vi "Configure Additional PUSCH Allocation.vi"(0 "VISA resource name":refnum<visa-resource-name>, 1 "DMRS Length (1)":i32=1, 2 "DMRS Power (0.0)":dbl format="%^.3e", 5 "Instance (1)":T3=1, 7 "Carrier Component (1)":T2=1, 9 "Allocation (1)":T1=1, 11 "error in (no error)":errorcluster, 12 "CDM Groups (1)":i32=1, 13 "Antenna Port (0)":i32) -> (4 "VISA resource name out":refnum<visa-resource-name>, 15 "error out":errorcluster)   [LabVIEW 2015, in "Rohde&Schwarz CMXP NR FR2 Measurement.lvlib"]
doc: "Specifies settings related to the PUSCH allocation, for carrier <no>, allocation <a>.\n\nAttribute:\nRSCMXPNRFR2M_ATTR_ADDITIONAL_PUSCH_ALLOCATION\n\nRemote-control command:\nCONFigure:NRMMw:MEAS<i>[:CC<no>]:ALLocation<a>:PUSCh:ADDitional"
uses:
  <instrlib>/Rohde&Schwarz CMXP NR FR2 Measurement/Rohde&Schwarz CMXP NR FR2 Measurement.lvlib
  <instrlib>/Rohde&Schwarz CMXP NR FR2 Measurement/Private/_Instance.ctl
  <instrlib>/Rohde&Schwarz CMXP NR FR2 Measurement/Private/_Carrier Component.ctl
  <instrlib>/Rohde&Schwarz CMXP NR FR2 Measurement/Private/_Allocation.ctl
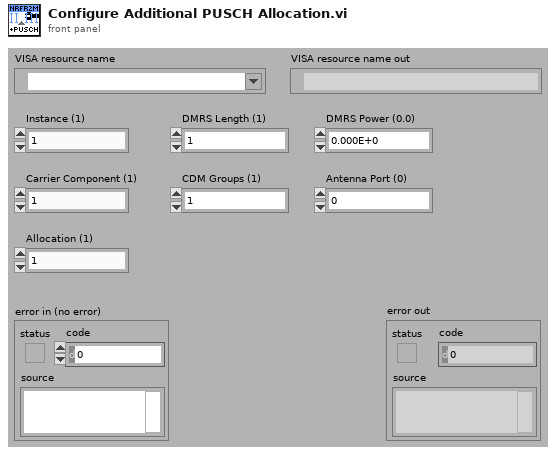
[diagram p1: front panel]
types:
  T1 = typedef "Rohde&Schwarz CMXP NR FR2 Measurement.lvlib/_Allocation.ctl" = i32
  T2 = typedef "Rohde&Schwarz CMXP NR FR2 Measurement.lvlib/_Carrier Component.ctl" = i32
  T3 = typedef "Rohde&Schwarz CMXP NR FR2 Measurement.lvlib/_Instance.ctl" = i32
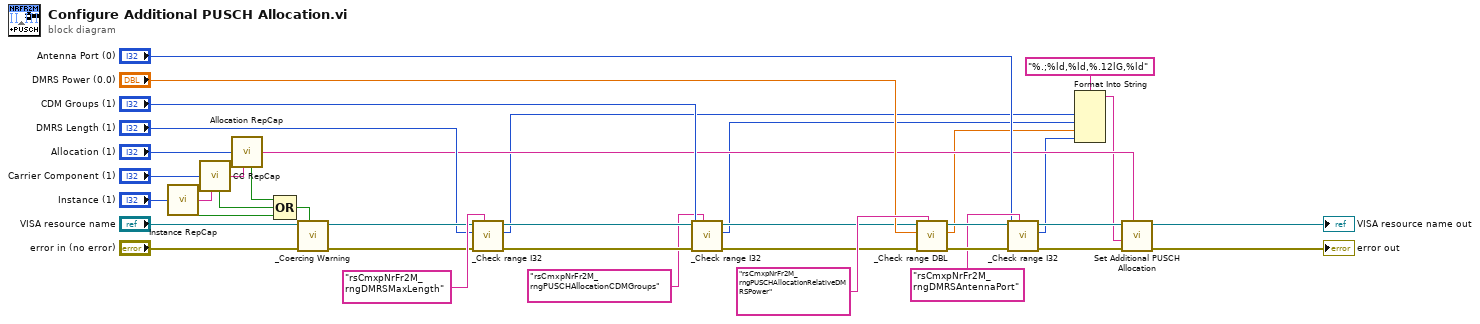
[diagram p0: block diagram]
diagram:
  n1 = call <instrlib>:"Instance RepCap.vi"("Instance In"="Instance (1)") -> ("In Range?"=w34:bool, "RepCap Identifier Out"=w2:string)  [unwired: 1 in]
  n2 = call <instrlib>:"CC RepCap.vi"("CC In"="Carrier Component (1)", "RepCap String In (\"\")"=w2) -> ("In Range?"=w33:bool, "RepCap Identifier Out"=w32:string)
  n3 = call <instrlib>:"Allocation RepCap.vi"("Allocation In"="Allocation (1)", "RepCap String In (\"\")"=w32) -> ("In Range?"=w31:bool, "RepCap Identifier Out"=w12:string)
  n4 = Compound Arithmetic op=OR(w31, w33, w34) -> (w36:bool)
  n5 = call <instrlib>:"_Coercing Warning.vi"("In Range?"=w36, "error in (no error)"="error in (no error)", "VISA resource name"="VISA resource name") -> ("error out"=w28:errorcluster, "VISA resource name out"=w27:refnum<visa-resource-name>)  [unwired: 7 in]
  n6 = call <instrlib>:"_Check range I32.vi"("Range Table Identifier"="rsCmxpNrFr2M_rngDMRSMaxLength", "error in (no error)"=w28, "I32 Value In"="DMRS Length (1)", "VISA resource name"=w27) -> ("error out"=w25:errorcluster, "I32 Value Out"=w7:i32, "VISA resource name out"=w24:refnum<visa-resource-name>)  [unwired: 5 in]
  n7 = call <instrlib>:"_Check range I32.vi"("Range Table Identifier"="rsCmxpNrFr2M_rngPUSCHAllocationCDMGroups", "error in (no error)"=w25, "I32 Value In"="CDM Groups (1)", "VISA resource name"=w24) -> ("error out"=w19:errorcluster, "I32 Value Out"=w6:i32, "VISA resource name out"=w18:refnum<visa-resource-name>)  [unwired: 5 in]
  n8 = call <instrlib>:"_Check range DBL.vi"("Range Table Identifier"="rsCmxpNrFr2M_rngPUSCHAllocationRelativeDMRSPower", "error in (no error)"=w19, "DBL Value In"="DMRS Power (0.0)", "VISA resource name"=w18) -> ("error out"=w16:errorcluster, "DBL Value Out"=w5:dbl, "VISA resource name out"=w17:refnum<visa-resource-name>)  [unwired: 5 in]
  n9 = call <instrlib>:"_Check range I32.vi"("Range Table Identifier"="rsCmxpNrFr2M_rngDMRSAntennaPort", "error in (no error)"=w16, "I32 Value In"="Antenna Port (0)", "VISA resource name"=w17) -> ("error out"=w10:errorcluster, "I32 Value Out"=w4:i32, "VISA resource name out"=w11:refnum<visa-resource-name>)  [unwired: 5 in]
  n10 = Format Into String(format string="%.;%ld,%ld,%.12lG,%ld", w7, w6, w5, w4) -> (resulting string=w1:string)  [unwired: 2 in, 1 out]
  n11 = call "Set Additional PUSCH Allocation"("Repeated Capabilities"=w12, "error in (no error)"=w10, "Additional PUSCH Allocation ()"=w1, "instrument handle"=w11) -> ("error out"=→"error out":errorcluster, "instrument handle out"=→"VISA resource name out":refnum<visa-resource-name>)  [unwired: 6 in]
